vi "SaveTune.vi"(0 "Array":dbl[](array[numeric]), 1 "Save Data to File":bool, 2 "Ext time (sec)":dbl format="%#_10g", 3 "RawSignal":dbl[](array[numeric])) -> ()   [LabVIEW 2018]
uses:
  Global 2.vi
  kleinjan/MKS/Global - Pressure & Flow.vi
  RunNumberGlobal.vi
panel:
  out "Error Message":string
  out "File name":string
  # "Saves data to spreadsheet file"
  # "Creates file with name including current time\nand header plus data"
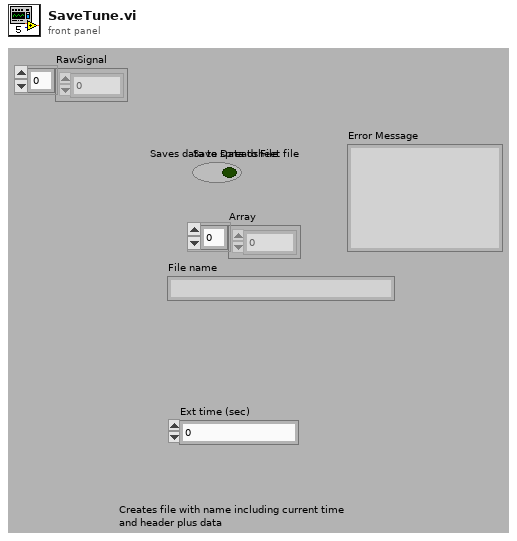
[diagram p1: front panel]
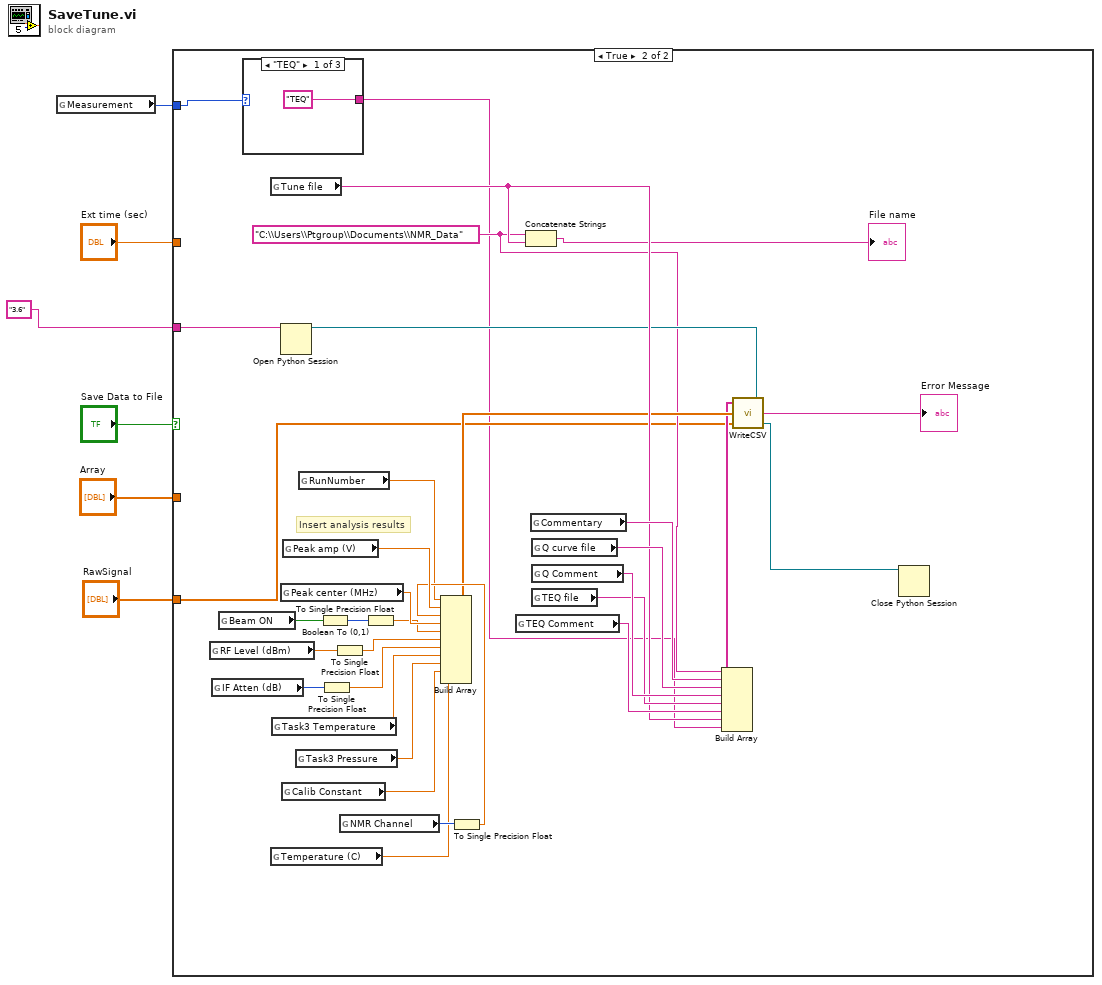
[diagram p0: block diagram]
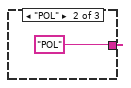
[diagram p3: hidden frame]
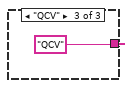
[diagram p4: hidden frame]
diagram:
  n1 = global read "Global 2.vi" "Measurement"() -> (w3:enum16{"TEQ", "POL", "QCV"})
  n2 = case shown="True" "Save Data to File" {
    tunnel: "Array" -> [_ _]
    tunnel: "Ext time (sec)" -> [_ _]
    tunnel: w3 -> [_ w11]
    tunnel: "3.6" ("Python version") -> [_ w17]
    tunnel: "RawSignal" -> [_ w12]
    frame False {
      # "Not writing file"
    }
    frame True {
      w13 = "C:\\Users\\Ptgroup\\Documents\\NMR_Data"
      # "Insert analysis results"
      n3 = global read "Global 2.vi" "RF Level (dBm)"() -> (w27:dbl)
      n4 = global read "Global 2.vi" "IF Atten (dB)"() -> (w25:i8)
      n5 = global read "Global 2.vi" "Beam ON"() -> (w29:bool)
      n6 = case shown="\"TEQ\"" w11 {
        tunnel: ["TEQ" "POL" "QCV"] -> w10
        frame "TEQ" {
        }
        frame "POL" {
        }
        frame "QCV" {
        }
      }
      n7 = global read "Global 2.vi" "Tune file"() -> (w21:string)
      n8 = global read "Global 2.vi" "Temperature (C)"() -> (w8:dbl)
      n9 = global read "Global - Pressure & Flow.vi" "Task3 Temperature"() -> (w23:dbl)
      n10 = Open Python Session(python version=w17) -> (session out=w16:refnum<k35>)  [unwired: 2 in, 1 out]
      n11 = global read "Global 2.vi" "Peak center (MHz)"() -> (w33:sgl)
      n12 = global read "Global 2.vi" "Calib Constant"() -> (w9:dbl)
      n13 = global read "Global 2.vi" "Peak amp (V)"() -> (w34:sgl)
      n14 = global read "Global - Pressure & Flow.vi" "Task3 Pressure"() -> (w22:dbl)
      n15 = global read "RunNumberGlobal.vi" "RunNumber"() -> (w7:dbl)
      n16 = Boolean To (0,1)(Boolean=w29) -> (0, 1=w30:i16)
      n17 = To Single Precision Float(number=w25) -> (single precision float=w24:sgl)
      n18 = To Single Precision Float(number=w27) -> (single precision float=w26:sgl)
      n19 = global read "Global 2.vi" "NMR Channel"() -> (w32:i32)
      n20 = To Single Precision Float(number=w30) -> (single precision float=w28:sgl)
      n21 = To Single Precision Float(number=w32) -> (single precision float=w31:sgl)
      n22 = Build Array(w7, w34, w31, w33, w28, w26, w24, w23, w22, w9, w8) -> (w20:dbl[])
      n23 = global read "Global 2.vi" "TEQ Comment"() -> (w36:string)
      n24 = Concatenate Strings(w13, w21) -> (→"File name":string)
      n25 = global read "Global 2.vi" "Commentary"() -> (w39:string)
      n26 = global read "Global 2.vi" "Q curve file"() -> (w38:string)
      n27 = global read "Global 2.vi" "Q Comment"() -> (w37:string)
      n28 = global read "Global 2.vi" "TEQ file"() -> (w35:string)
      n29 = Build Array(w13, w39, w38, w37, w35, w36, w21, w10) -> (w19:string[])
      n30 = call "WriteCSV.vi"("session in"=w16, "Signal"=w12, "NumericData"=w20, "StringData"=w19) -> ("session out"=w15:refnum<k35>, "Error Message"=→"Error Message":string)
      n31 = Close Python Session(session in=w15) -> ()  [unwired: 1 in, 1 out]
    }
  }
